vi "Load Category Totals.vi"(8 "error in (no error)":errorcluster, 11 "Budgetizer in":refnum<class "Budgetizer.lvclass">) -> (0 "error out":errorcluster, 3 "Budgetizer out":refnum<class "Budgetizer.lvclass">)   [LabVIEW 2018, in "Budgetizer.lvclass"]
uses:
  Budgetizer.lvclass
  Budgetizer.lvclass/Budgetizer.ctl
  database/Database.lvclass
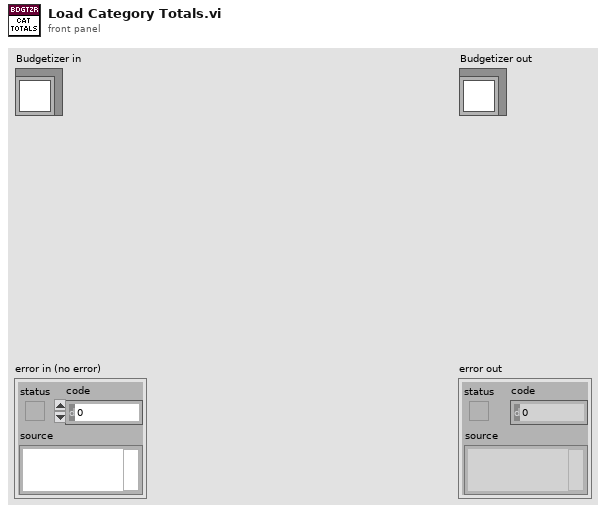
[diagram p1: front panel]
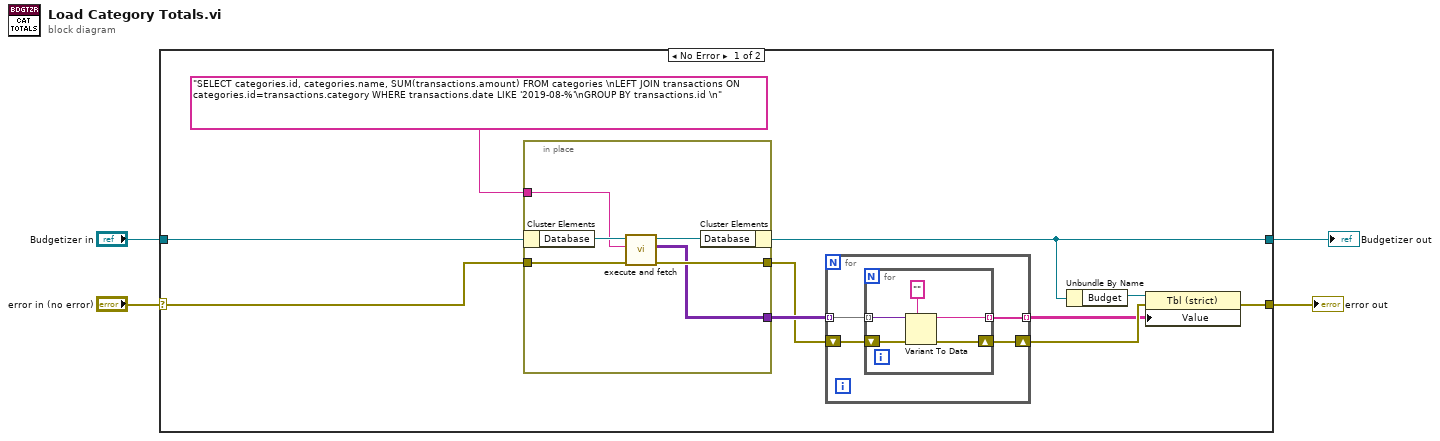
[diagram p0: block diagram]
diagram:
  n1 = case shown="No Error" "error in (no error)" {
    selector: "error in (no error)" -> [w13 w31]
    tunnel: [w6 w31] -> w3
    tunnel: [w10 w30] -> w1
    tunnel: "Budgetizer in" -> [w14 w30]
    frame No Error {
      n2 = in-place {
        in-place-border: w13 -> [w27]
        in-place-border: [w26] -> w11
        in-place-border: "SELECT categories.id, categories.name, SUM(transactions.amount) FROM categories \nLEFT JOIN transactions ON categories.id=transactions.category WHERE transactions.date LIKE '2019-08-%'\nGROUP BY transactions.id \n" -> [w25]
        in-place-border: [w24] -> w12
        n3 = in-place-cluster #1(w14) -> ("Database"=w29:refnum<class "Database.lvclass">)
        n4 = call "execute and fetch.vi"("error in (no error)"=w27, "SQL query"=w25, "Database in"=w29) -> ("error out"=w26:errorcluster, "recordset data"=w24:variant[][], "Database out"=w28:refnum<class "Database.lvclass">)  [unwired: 5 in, 1 out]
        n5 = in-place-cluster #1("Database"=w28) -> (w10:refnum<class "Budgetizer.lvclass">)
      }
      n6 = for {
        tunnel: w12 -> [w18] mode=indexing
        shift-right: [w16] -> w8
        shift-left: w11 -> [w17]
        tunnel: [w15] -> w7 mode=indexing
        n7 = for {
          tunnel: w18 -> [w23] mode=indexing
          shift-right: [w21] -> w16
          shift-left: w17 -> [w22]
          tunnel: [w19] -> w15 mode=indexing
          n8 = Variant To Data(error in=w22, type="", Variant=w23) -> (data=w19:string, error out=w21:errorcluster)
        }
      }
      n9 = Unbundle By Name(w10) -> ("Budget"=w9:refnum<vi>)
      n10 = property class="Tbl (strict)"(reference=w9, error in=w8, "Value"=w7) -> (error out=w6:errorcluster)  [unwired: 1 out]
    }
    frame Error {
    }
  }
  "error out" <- w3
  "Budgetizer out" <- w1
